vi "cvt.vi"(7 "LVWSR":refnum<class "Web Request.lvclass">, 11 "force":u8) -> ()   [LabVIEW 2017]
uses:
  <vilib>/wsapi/Web Request.lvclass
  Controller/gController.lvclass
panel:
  out "String":string
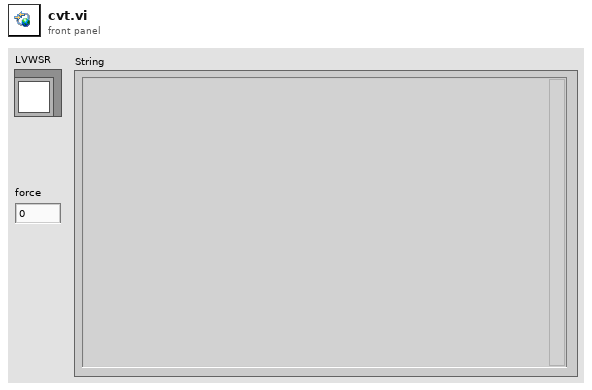
[diagram p1: front panel]
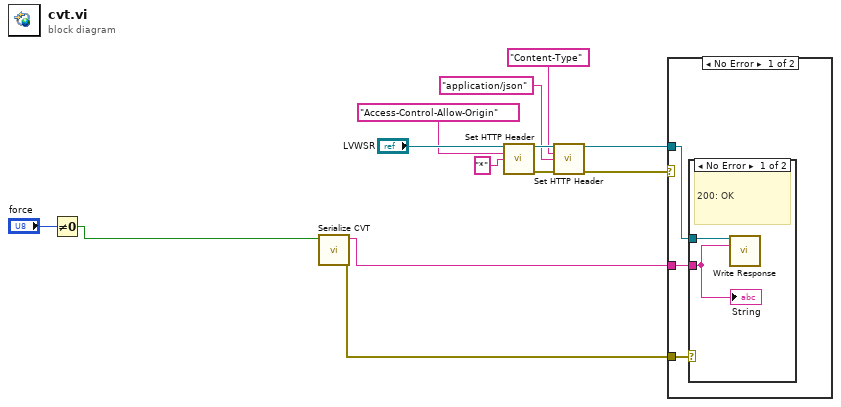
[diagram p0: block diagram]
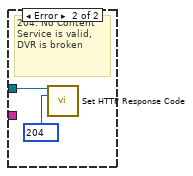
[diagram p2: hidden frame]
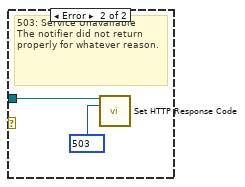
[diagram p3: hidden frame]
diagram:
  n1 = Not Equal To 0?(x="force") -> (x != 0?=w3:bool)
  n2 = call "Serialize CVT.vi"("force?"=w3) -> ("error out"=w1:errorcluster, "json out"=w2:string)  [unwired: 9 in]
  n3 = call <vilib>:"Set HTTP Header.vi"("LabVIEW Web Service Request"="LVWSR", "header"="Access-Control-Allow-Origin", "header value"="*") -> ("LabVIEW Web Service Request out"=w12:refnum<class "Web Request.lvclass">, "error out"=w11:errorcluster)  [unwired: 11 in]
  n4 = call <vilib>:"Set HTTP Header.vi"("LabVIEW Web Service Request"=w12, "header"="Content-Type", "header value"="application/json", "error in (no error)"=w11) -> ("LabVIEW Web Service Request out"=w8:refnum<class "Web Request.lvclass">, "error out"=w7:errorcluster)  [unwired: 10 in]
  n5 = case shown="No Error" w7 {
    tunnel: w1 -> [w16 _]
    tunnel: w8 -> [w15 w22]
    tunnel: w2 -> [w14 _]
    frame No Error {
      n6 = case shown="No Error" w16 {
        tunnel: w15 -> [w18 w20]
        tunnel: w14 -> [w17 _]
        frame No Error {
          # "200: OK"
          n7 = call <vilib>:"Write Response.vi"("LabVIEW Web Service Request"=w18, "response string"=w17) -> ()  [unwired: 12 in, 2 out]
          "String" <- w17
        }
        frame Error {
          w19 = 204 items=["100"=100, "101"=101, "200"=200, "201"=201, "202"=202, "203"=203, "204"=204, "205"=205, "206"=206, "300"=300, "301"=301, "302"=302, "303"=303, "304"=304, "305"=305, "306"=306, "307"=307, "400"=400, "401"=401, "402"=402, "403"=403, "404"=404, "405"=405, "406"=406, "407"=407, "408"=408, "409"=409, "410"=410, "411"=411, "412"=412, "413"=413, "414"=414, "415"=415, "416"=416, "417"=417, "500"=500, "501"=501, "502"=502, "503"=503, "504"=504, "505"=505] ("response code (200)")
          # "204: No Content\nService is valid, DVR is broken"
          n8 = call <vilib>:"Set HTTP Response Code.vi"("LabVIEW Web Service Request"=w20, "response code (200)"=w19) -> ()  [unwired: 12 in, 2 out]
        }
      }
    }
    frame Error {
      w21 = 503 items=["100"=100, "101"=101, "200"=200, "201"=201, "202"=202, "203"=203, "204"=204, "205"=205, "206"=206, "300"=300, "301"=301, "302"=302, "303"=303, "304"=304, "305"=305, "306"=306, "307"=307, "400"=400, "401"=401, "402"=402, "403"=403, "404"=404, "405"=405, "406"=406, "407"=407, "408"=408, "409"=409, "410"=410, "411"=411, "412"=412, "413"=413, "414"=414, "415"=415, "416"=416, "417"=417, "500"=500, "501"=501, "502"=502, "503"=503, "504"=504, "505"=505] ("response code (200)")
      # "503: Service Unavailable\nThe notifier did not return properly for whatever reason."
      n9 = call <vilib>:"Set HTTP Response Code.vi"("LabVIEW Web Service Request"=w22, "response code (200)"=w21) -> ()  [unwired: 12 in, 2 out]
    }
  }
